vi "AlazarFFTBackgroundSubtractionSetEnabled.vi"(3 "error in (no error)":errorcluster, 4 "Enabled":u32 format="%.0g", 5 "DSP Handle":u64) -> (0 "error out":errorcluster, 1 "Return Code":u32, 2 "DSP Handle":u64)   [LabVIEW 2018]
uses:
  ATSApi.dll
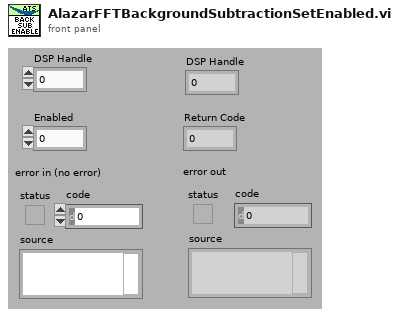
[diagram p1: front panel]
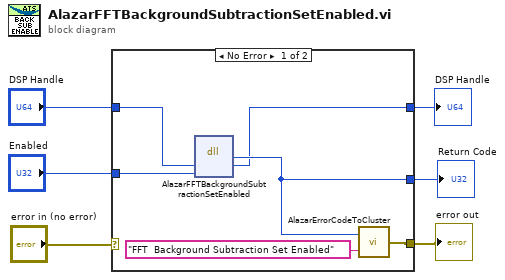
[diagram p0: block diagram]
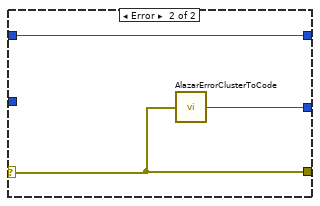
[diagram p2: hidden frame]
diagram:
  n1 = case shown="No Error" "error in (no error)" {
    selector: "error in (no error)" -> [_ w14]
    tunnel: [w10 w14] -> w4
    tunnel: [w12 w15] -> w3
    tunnel: [w9 w13] -> w5
    tunnel: "Enabled" -> [w8 _]
    tunnel: "DSP Handle" -> [w7 w13]
    frame No Error {
      n2 = dll-call lib="ATSApi.dll" fn="AlazarFFTBackgroundSubtractionSetEnabled"("dspHandle"=w7, "enabled"=w8) -> ("return type"=w12:u32, "dspHandle"=w9:u64)  [unwired: 4 in, 2 out]
      n3 = call "AlazarErrorCodeToCluster.vi"("Message"="FFT  Background Subtraction Set Enabled", "Error Code"=w12) -> ("error out"=w10:errorcluster)
    }
    frame Error {
      n4 = call "AlazarErrorClusterToCode.vi"("error in (no error)"=w14) -> ("Error Code"=w15:u32)
    }
  }
  "DSP Handle" <- w5
  "error out" <- w4
  "Return Code" <- w3
